vi "1.0 Producer Consumer Test.vi"() -> ()   [LabVIEW 2018]
uses:
  <vilib>/DAQmx/read.llb/DAQmx Read (Analog Wfm 1Chan 1Samp).vi
  <vilib>/DAQmx/create/channels.llb/DAQmx Create Channel (AI-Voltage-Basic).vi
  <vilib>/DAQmx/configure/timing.llb/DAQmx Timing (Sample Clock).vi
  <vilib>/DAQmx/miscellaneous.llb/DAQmx Fill In Error Info.vi
panel:
  out "Numeric 2":dbl
  out "Numeric":dbl
  in  "stop":bool
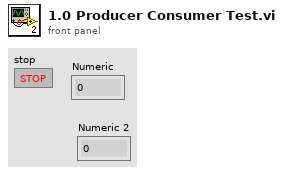
[diagram p1: front panel]
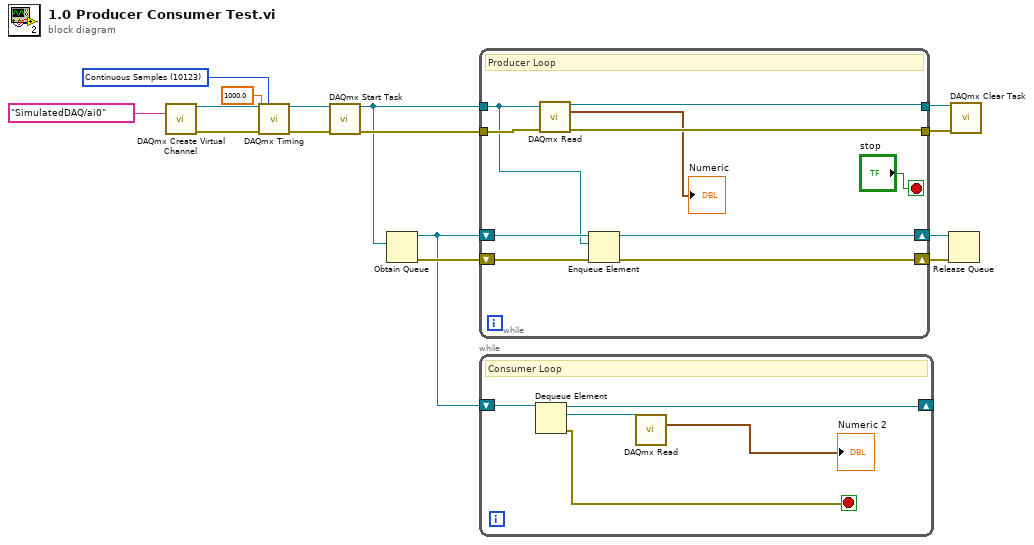
[diagram p0: block diagram]
diagram:
  w11 = 10123 items=["Finite Samples"=10178, "Continuous Samples"=10123, "Hardware Timed Single Point"=12522] ("sample mode")
  n1 = call-poly <vilib>:"DAQmx Create Virtual Channel.vi"("physical channels"=tag "SimulatedDAQ/ai0") -> ("task out"=w12:refnum<k21>, "error out"=w13:errorcluster)  [unwired: 13 in]
  n2 = call-poly <vilib>:"DAQmx Timing.vi"("task/channels in"=w12, "sample mode"=w11, "rate"=1000.0, "error in"=w13) -> ("task out"=w14:refnum<k21>, "error out"=w15:errorcluster)  [unwired: 10 in]
  n3 = call <vilib>:"DAQmx Start Task.vi"("task/channels in"=w14, "error in"=w15) -> ("task out"=w2:refnum<k21>, "error out"=w3:errorcluster)  [unwired: 12 in]
  n4 = Obtain Queue(element data type=w2) -> (queue out=w1:refnum<queue>, error out=w6:errorcluster)  [unwired: 4 in, 1 out]
  n5 = while {
    tunnel: w2 -> [w17]
    tunnel: w3 -> [w24]
    tunnel: [w23] -> w9
    tunnel: [w22] -> w8
    shift-right: [w19] -> w5
    shift-left: w1 -> [w21]
    shift-right: [w18] -> w4
    shift-left: w6 -> [w20]
    stop <- "stop" stop-if-true
    # "Producer Loop"
    n6 = call-poly <vilib>:"DAQmx Read.vi"("task/channels in"=w17, "error in"=w24) -> ("task out"=w23:refnum<k21>, "data"=→"Numeric":waveform(dbl), "error out"=w22:errorcluster)  [unwired: 11 in]
    n7 = Enqueue Element(queue=w21, element=w17, error in (no error)=w20) -> (queue out=w19:refnum<queue>, error out=w18:errorcluster)  [unwired: 1 in, 1 out]
  }
  n8 = while {
    shift-right: [w29] -> _
    shift-left: w1 -> [w30]
    stop <- w28 stop-if-true
    # "Consumer Loop"
    n9 = Dequeue Element(queue=w30) -> (queue out=w29:refnum<queue>, element=w27:refnum<k21>, error out=w28:errorcluster)  [unwired: 2 in, 1 out]
    n10 = call-poly <vilib>:"DAQmx Read.vi"("task/channels in"=w27) -> ("data"=→"Numeric 2":waveform(dbl))  [unwired: 12 in, 2 out]
  }
  n11 = Release Queue(queue=w5, error in (no error)=w4) -> ()  [unwired: 1 in, 3 out]
  n12 = call <vilib>:"DAQmx Clear Task.vi"("task in"=w9, "error in"=w8) -> ()  [unwired: 13 in, 1 out]
